vi "Set_BSA_Coincidence.vi"(0 "GPIB address":string, 2 "Set Coincidence":enum16{"Slave", "Master", "Private"}(ring)=enum."Master", 3 "error in (no error)":errorcluster) -> (6 "Coincidence Read":enum16{"Slave", "Master", "Private"}(ring)=enum."Master", 7 "error out":errorcluster)   [LabVIEW 2010]
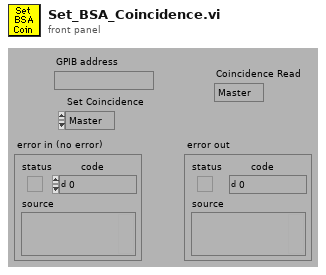
[diagram p1: front panel]
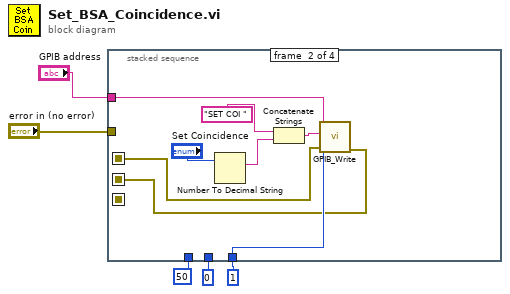
[diagram p0: block diagram]
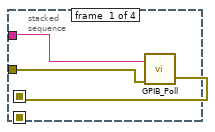
[diagram p2: hidden frame]
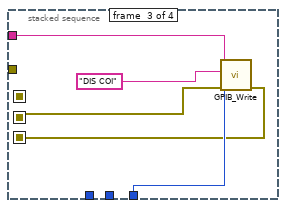
[diagram p3: hidden frame]
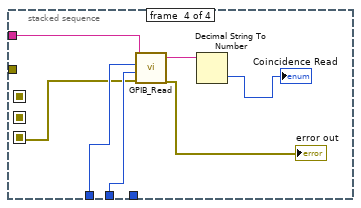
[diagram p4: hidden frame]
diagram:
  n1 = stacked-sequence {
    seq-local: [w6 _ _ _] -> [_ w11 _ _]
    seq-local: [_ w10 _ _] -> [_ _ w18 _]
    seq-local: [_ _ w17 _] -> [_ _ _ w24]
    tunnel: "GPIB address" -> [w8 w16 w21 w28]
    tunnel: 1 -> [_ w15 w20 _]
    tunnel: 0 -> [_ _ _ w27]
    tunnel: 50 -> [_ _ _ w26]
    tunnel: "error in (no error)" -> [w7 _ _ _]
    frame #0 {
      n2 = call "GPIB_Poll.vi"("error in"=w7, "address string"=w8) -> ("error out"=w6:errorcluster)  [unwired: 1 out]
    }
    frame #1 {
      n3 = Number To Decimal String(number="Set Coincidence") -> (decimal integer string=w14:string)  [unwired: 1 out]
      n4 = Concatenate Strings("SET COI ", w14) -> (w12:string)
      n5 = call "GPIB_Write.vi"("address string"=w16, "data In"=w12, "mode (0)"=w15, "error in"=w11) -> ("error out"=w10:errorcluster)  [unwired: 1 in, 1 out]
    }
    frame #2 {
      n6 = call "GPIB_Write.vi"("address string"=w21, "data In"="DIS COI", "mode (0)"=w20, "error in"=w18) -> ("error out"=w17:errorcluster)  [unwired: 1 in, 1 out]
    }
    frame #3 {
      n7 = call "GPIB_Read.vi"("address string"=w28, "byte count"=w26, "mode (0)"=w27, "error in"=w24) -> ("data Out"=w25:string, "error out"=→"error out":errorcluster)  [unwired: 1 in, 1 out]
      n8 = Decimal String To Number(string=w25) -> (number=→"Coincidence Read":i32)  [unwired: 3 out]
    }
  }
